vi "Acquire.vi"(8 "error in (no error)":errorcluster, 9 "Data Queue":refnum<queue>, 10 "Data Notifier":refnum<notifier>, 11 "Hardware Resources in":T1={"VISA resource name"="", "DAQ Type"=0, "Channel 1"={"Acquiring"=FALSE, "Enabled"=FALSE, "Terminal configuration"=32767, "Range"=0, "Coupling"=0}, "Channel 2"={"Acquiring"=FALSE, "Enabled"=FALSE, "Terminal configuration"=0, "Range"=0, "Coupling"=0}, "Timing"={"Sample Time [Time Units]"=0, "Actual Sample Time [s]"=0.0, "Samples per Iteration"=0, "Sample Clock Source"=0, "Time Units"=0, "t0"=timestamp(0 s since 1904-01-01), "Baud rate"=0}, "PS Parameters"={"PS handle"=0, "PS Max_adc"=32767, "PS Enabled Array"=[], "PS Device Info"={"Driver Version"="", "USB Version"="", "Hardware"="", "Variant"="", "Batch and Serial"="", "Cal Date"="", "Kernel Version"="", "Digital HW Version"="", "Analogue HW Version"="", "Firmware 1"="", "Firmware 2"="", "MSO"=FALSE, "Number of Channels"=0}, "Channel 1 Buffer"=refnum, "Channel 2 Buffer"=refnum, "Resolution"=0, "USB Power"=FALSE}, "Trigger"={"Direction"=0, "Threshold [V]"=0.0, "Enabled"=FALSE, "Trigger Source"=0}, "Keithley Parameters"={"Previous End / Current Start"=0, "Quantity"=0}} {"Keithley Parameters"."Quantity" items=["Current", "Voltage"]; "Trigger"."Trigger Source" items=["Channel 1"=0, "Channel 2"=1, "Ext."=4]; "Trigger"."Direction" items=["Falling", "Rising"]; "PS Parameters"."Resolution" items=["8", "12", "14", "15", "16"]; "Timing"."Time Units" items=["Seconds"]; "Timing"."Sample Clock Source" items=["Internal", "External"]; "Channel 2"."Coupling" items=["AC", "DC"]; "Channel 2"."Range" items=["0.01", "0.02", "0.05", "0.1", "0.2", "0.5", "1", "2", "5", "10", "20", "50", "100", "1000"]; "Channel 2"."Terminal configuration" items=["Referenced Single Ended", "Differential"]; "Channel 1"."Coupling" items=["AC", "DC"]; "Channel 1"."Range" items=["0.01", "0.02", "0.05", "0.1", "0.2", "0.5", "1", "2", "5", "10", "20", "50", "100", "1000"]; "Channel 1"."Terminal configuration" items=["Referenced Single Ended", "Differential"]; "DAQ Type" items=["Simulated", "Tektronics DPO2k/3k/4k", "PicoScope 2000a Series", "Keithley DMM7510", "PicoScope 5000a Series", "Arduino"]}) -> (0 "error out":errorcluster, 3 "Hardware Resources out":T1={"VISA resource name"="", "DAQ Type"=0, "Channel 1"={"Acquiring"=FALSE, "Enabled"=FALSE, "Terminal configuration"=32767, "Range"=0, "Coupling"=0}, "Channel 2"={"Acquiring"=FALSE, "Enabled"=FALSE, "Terminal configuration"=0, "Range"=0, "Coupling"=0}, "Timing"={"Sample Time [Time Units]"=0, "Actual Sample Time [s]"=0.0, "Samples per Iteration"=0, "Sample Clock Source"=0, "Time Units"=0, "t0"=timestamp(0 s since 1904-01-01), "Baud rate"=0}, "PS Parameters"={"PS handle"=0, "PS Max_adc"=32767, "PS Enabled Array"=[], "PS Device Info"={"Driver Version"="", "USB Version"="", "Hardware"="", "Variant"="", "Batch and Serial"="", "Cal Date"="", "Kernel Version"="", "Digital HW Version"="", "Analogue HW Version"="", "Firmware 1"="", "Firmware 2"="", "MSO"=FALSE, "Number of Channels"=0}, "Channel 1 Buffer"=refnum, "Channel 2 Buffer"=refnum, "Resolution"=0, "USB Power"=FALSE}, "Trigger"={"Direction"=0, "Threshold [V]"=0.0, "Enabled"=FALSE, "Trigger Source"=0}, "Keithley Parameters"={"Previous End / Current Start"=0, "Quantity"=0}} {"Keithley Parameters"."Quantity" items=["Current", "Voltage"]; "Trigger"."Trigger Source" items=["Channel 1"=0, "Channel 2"=1, "Ext."=4]; "Trigger"."Direction" items=["Falling", "Rising"]; "PS Parameters"."Resolution" items=["8", "12", "14", "15", "16"]; "Timing"."Time Units" items=["Seconds"]; "Timing"."Sample Clock Source" items=["Internal", "External"]; "Channel 2"."Coupling" items=["AC", "DC"]; "Channel 2"."Range" items=["0.01", "0.02", "0.05", "0.1", "0.2", "0.5", "1", "2", "5", "10", "20", "50", "100", "1000"]; "Channel 2"."Terminal configuration" items=["Referenced Single Ended", "Differential"]; "Channel 1"."Coupling" items=["AC", "DC"]; "Channel 1"."Range" items=["0.01", "0.02", "0.05", "0.1", "0.2", "0.5", "1", "2", "5", "10", "20", "50", "100", "1000"]; "Channel 1"."Terminal configuration" items=["Referenced Single Ended", "Differential"]; "DAQ Type" items=["Simulated", "Tektronics DPO2k/3k/4k", "PicoScope 2000a Series", "Keithley DMM7510", "PicoScope 5000a Series", "Arduino"]})   [LabVIEW 2017, in "Acquisition.lvlib"]
doc: "Perform the acquisition. Replace the contents of this diagram with calls to acquisition hardware."
uses:
  Acquisition.lvlib
  Hardware Configuration.ctl
  Signal Type.ctl
  Settings/Terminal Configuration.ctl
  Settings/Range.ctl
  Settings/Coupling.ctl
  Settings/Sampling Clock Source.ctl
  Settings/Time Units.ctl
  Settings/Resolution.ctl
  Settings/Trigger Direction.ctl
  Settings/Trigger Source.ctl
  Settings/Quantity.ctl
  support/Active channels.vi
  Settings/Settings.lvlib
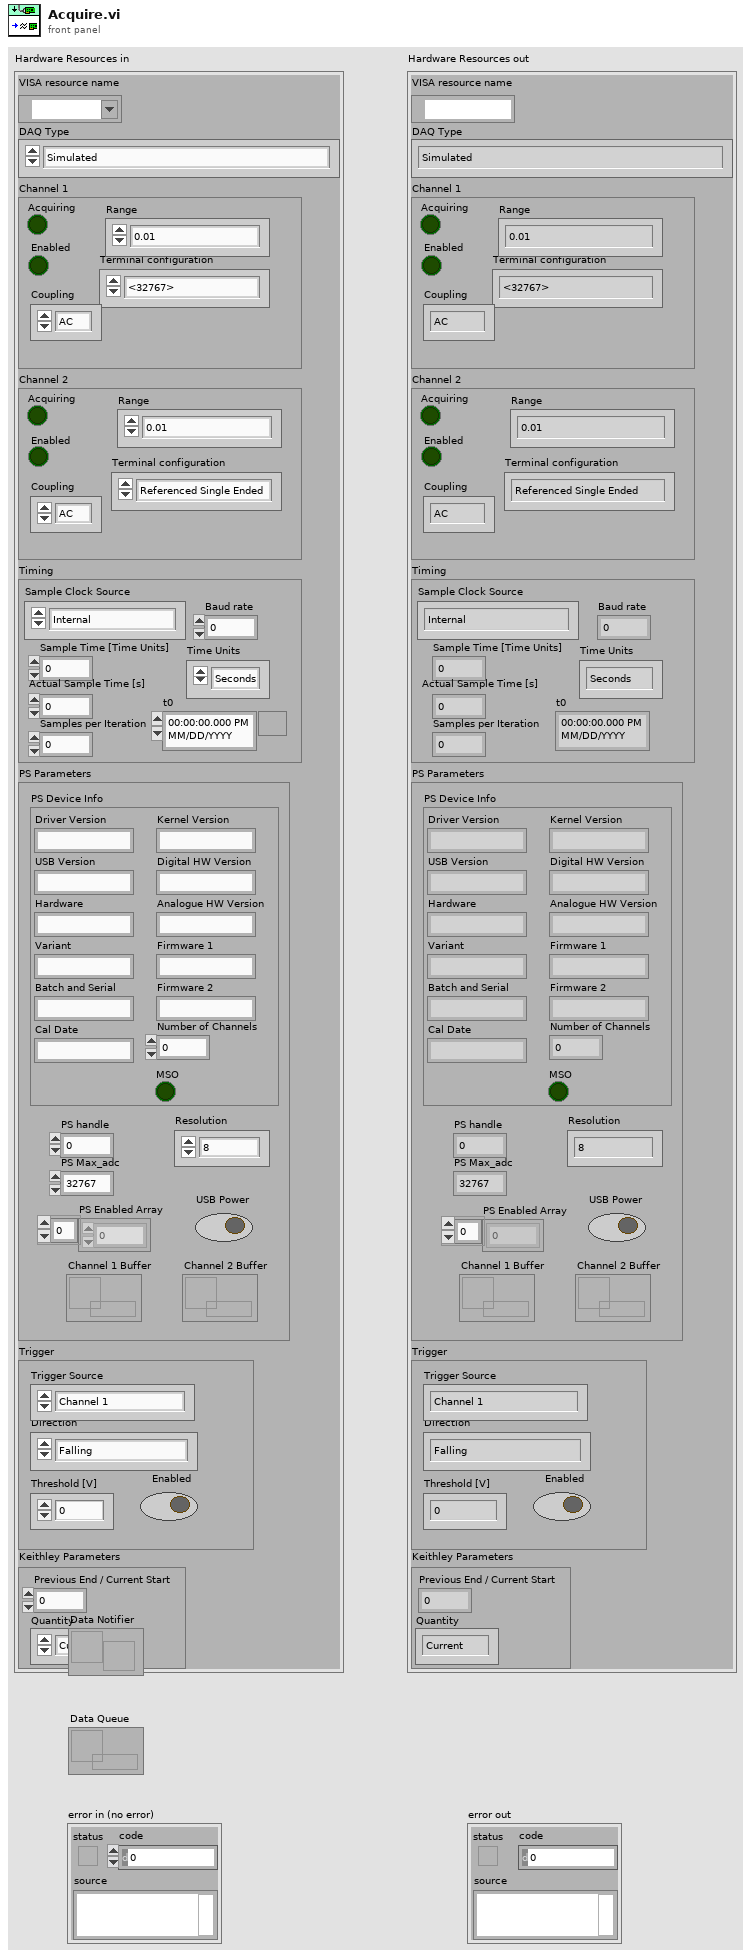
[diagram p1: front panel]
types:
  T1 = typedef "Acquisition.lvlib/Hardware Configuration.ctl" = cluster{"VISA resource name":refnum<visa-resource-name>, "DAQ Type":T2, "Channel 1":cluster{"Acquiring":bool, "Enabled":bool, "Terminal configuration":T3, "Range":T4, "Coupling":T5}, "Channel 2":cluster{"Acquiring":bool, "Enabled":bool, "Terminal configuration":T3, "Range":T4, "Coupling":T5}, "Timing":cluster{"Sample Time [Time Units]":u32, "Actual Sample Time [s]":dbl, "Samples per Iteration":u32, "Sample Clock Source":T6, "Time Units":T7, "t0":timestamp, "Baud rate":u32}, "PS Parameters":cluster{"PS handle":i16, "PS Max_adc":i16, "PS Enabled Array":i16[], "PS Device Info":cluster{"Driver Version":string, "USB Version":string, "Hardware":string, "Variant":string, "Batch and Serial":string, "Cal Date":string, "Kernel Version":string, "Digital HW Version":string, "Analogue HW Version":string, "Firmware 1":string, "Firmware 2":string, "MSO":bool, "Number of Channels":i16}, "Channel 1 Buffer":refnum<data-value>, "Channel 2 Buffer":refnum<data-value>, "Resolution":T8, "USB Power":bool}, "Trigger":cluster{"Direction":T9, "Threshold [V]":dbl, "Enabled":bool, "Trigger Source":T10}, "Keithley Parameters":cluster{"Previous End / Current Start":i32, "Quantity":T11}}
  T2 = typedef "Acquisition.lvlib/Signal Type.ctl" = u16
  T3 = typedef "Settings.lvlib/Terminal Configuration.ctl" = u16
  T4 = typedef "Settings.lvlib/Range.ctl" = u16
  T5 = typedef "Settings.lvlib/Coupling.ctl" = i16
  T6 = typedef "Settings.lvlib/Sampling Clock Source.ctl" = u16
  T7 = typedef "Settings.lvlib/Time Units.ctl" = u32
  T8 = typedef "Settings.lvlib/Resolution.ctl" = i32
  T9 = typedef "Settings.lvlib/Trigger Direction.ctl" = u16
  T10 = typedef "Settings.lvlib/Trigger Source.ctl" = u16
  T11 = typedef "Settings.lvlib/Quantity.ctl" = u16
  T12 = cluster{"PS handle":i16, "PS Max_adc":i16, "PS Enabled Array":i16[], "PS Device Info":cluster{"Driver Version":string, "USB Version":string, "Hardware":string, "Variant":string, "Batch and Serial":string, "Cal Date":string, "Kernel Version":string, "Digital HW Version":string, "Analogue HW Version":string, "Firmware 1":string, "Firmware 2":string, "MSO":bool, "Number of Channels":i16}, "Channel 1 Buffer":refnum<data-value>, "Channel 2 Buffer":refnum<data-value>, "Resolution":T8, "USB Power":bool}
  T13 = cluster{"Previous End / Current Start":i32, "Quantity":T11}
  T14 = cluster{"Acquiring":bool, "Enabled":bool, "Terminal configuration":T3, "Range":T4, "Coupling":T5}
  T15 = cluster{"Sample Time [Time Units]":u32, "Actual Sample Time [s]":dbl, "Samples per Iteration":u32, "Sample Clock Source":T6, "Time Units":T7, "t0":timestamp, "Baud rate":u32}
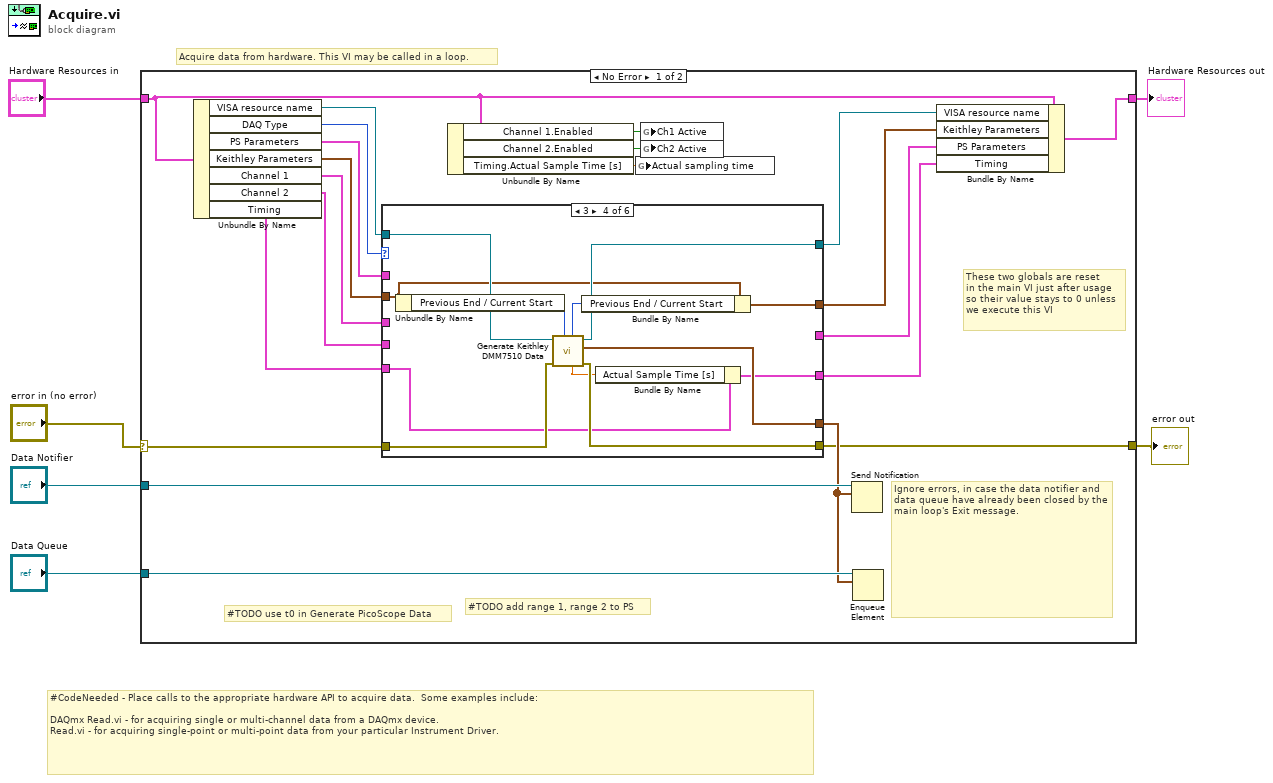
[diagram p0: block diagram]
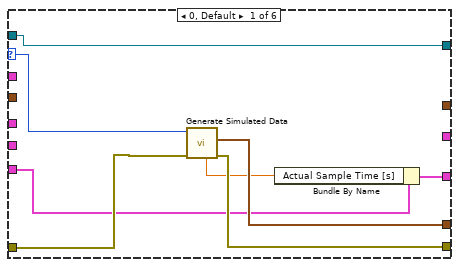
[diagram p2: hidden frame]
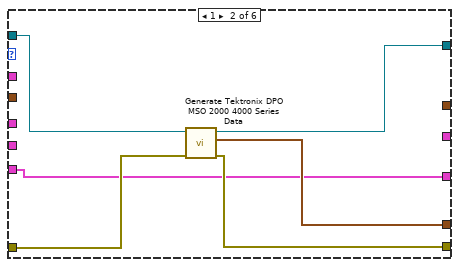
[diagram p3: hidden frame]
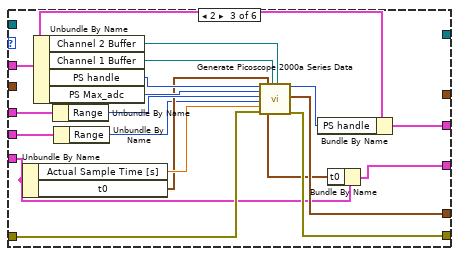
[diagram p4: hidden frame]
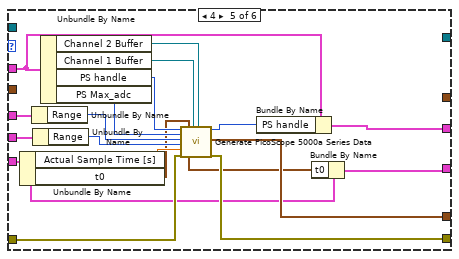
[diagram p5: hidden frame]
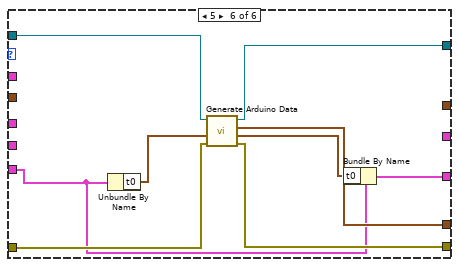
[diagram p6: hidden frame]
diagram:
  # "Acquire data from hardware. This VI may be called in a loop."
  # "#CodeNeeded - Place calls to the appropriate hardware API to acquire data.  Some examples include:\n\nDAQmx Read.vi - for acquiring single or multi-channel data from a DAQmx device.\nRead.vi - for acquiring single-point or multi-point data from your particular Instrument Driver."
  n1 = case shown="No Error" "error in (no error)" {
    selector: "error in (no error)" -> [w26 w101]
    tunnel: [w22 w101] -> w5
    tunnel: "Hardware Resources in" -> [w10 w102]
    tunnel: [w27 w102] -> w3
    tunnel: "Data Notifier" -> [w25 _]
    tunnel: "Data Queue" -> [w24 _]
    frame No Error {
      # "#TODO add range 1, range 2 to PS"
      # "These two globals are reset\nin the main VI just after usage\nso their value stays to 0 unless\nwe execute this VI"
      # "#TODO use t0 in Generate PicoScope Data"
      # "Ignore errors, in case the data notifier and data queue have already been closed by the main loop's Exit message."
      n2 = Unbundle By Name(w10) -> ("VISA resource name"=w20:refnum<visa-resource-name>, "DAQ Type"=w21:T2, "PS Parameters"=w15:T12, "Keithley Parameters"=w18:T13, "Channel 1"=w14:T14, "Channel 2"=w13:T14, "Timing"=w12:T15)
      n3 = case shown="3" w21 {
        selector: w21 -> [w31 _ _ _ _ _]
        tunnel: w26 -> [w34 w41 w59 w71 w91 w99]
        tunnel: [w32 w38 w55 w68 w89 w97] -> w23
        tunnel: [w33 w40 w58 w69 w90 w98] -> w22
        tunnel: w20 -> [w35 w39 _ w72 _ w100]
        tunnel: [w35 w37 _ w70 _ w96] -> w19
        tunnel: w18 -> [_ _ _ w66 _ _]
        tunnel: w15 -> [_ _ w57 _ w87 _]
        tunnel: w12 -> [w30 w36 w45 w63 w76 w93]
        tunnel: [_ _ w60 _ w85 _] -> w17
        tunnel: [_ _ _ w64 _ _] -> w16
        tunnel: w14 -> [_ _ w50 _ w80 _]
        tunnel: w13 -> [_ _ w49 _ w78 _]
        tunnel: [w29 w36 w43 w61 w75 w92] -> w11
        frame 0, Default {
          n4 = call "Generate Simulated Data.vi"("error in (no error)"=w34, "Signal Type"=w31) -> ("error out"=w33:errorcluster, "Graph Data"=w32:waveform(dbl)[], "Sampling time"=w28:dbl)  [unwired: 7 in]
          n5 = Bundle By Name(cluster=w30, "Actual Sample Time [s]"=w28) -> (w29:T15)
        }
        frame 1 {
          n6 = call "Generate Tektronix DPO MSO 2000 4000 Series Data.vi"("error in (no error)"=w41, "VISA resource name"=w39) -> ("error out"=w40:errorcluster, "Graph Data"=w38:waveform(dbl)[], "VISA resource name 2"=w37:refnum<visa-resource-name>)  [unwired: 7 in]
        }
        frame 2 {
          n7 = Unbundle By Name(w45) -> ("Actual Sample Time [s]"=w47:dbl, "t0"=w46:timestamp)
          n8 = Unbundle By Name(w57) -> ("Channel 2 Buffer"=w54:refnum<data-value>, "Channel 1 Buffer"=w53:refnum<data-value>, "PS handle"=w52:i16, "PS Max_adc"=w51:i16)
          n9 = Unbundle By Name(w50) -> ("Range"=w48:T4)
          n10 = Unbundle By Name(w49) -> ("Range"=w42:T4)
          n11 = call "Generate Picoscope 2000a Series Data.vi"("handle in"=w52, "Max ADC"=w51, "Ch1 Range Index"=w48, "Ch2 Range Index"=w42, "Actual Sample Interval"=w47, "error in (no error)"=w59, "t0"=w46, "Channel 1 Buff In"=w53, "Channel 2 Buff In"=w54) -> ("next t0"=w44:timestamp, "handle out"=w56:i16, "Graph Data"=w55:waveform(dbl)[], "error out"=w58:errorcluster)  [unwired: 5 in, 2 out]
          n12 = Bundle By Name(cluster=w57, "PS handle"=w56) -> (w60:T12)
          n13 = Bundle By Name(cluster=w45, "t0"=w44) -> (w43:T15)
        }
        frame 3 {
          n14 = Unbundle By Name(w66) -> ("Previous End / Current Start"=w67:i32)
          n15 = call "Generate Keithley DMM7510 Data.vi"("Previous End"=w67, "error in (no error)"=w71, "VISA resource name in"=w72) -> ("error out"=w69:errorcluster, "Graph Data"=w68:waveform(dbl)[], "VISA resource name out"=w70:refnum<visa-resource-name>, "Actual sampling time (mean)"=w62:dbl, "Current End"=w65:i32)  [unwired: 4 in]
          n16 = Bundle By Name(cluster=w66, "Previous End / Current Start"=w65) -> (w64:T13)
          n17 = Bundle By Name(cluster=w63, "Actual Sample Time [s]"=w62) -> (w61:T15)
        }
        frame 4 {
          n18 = Unbundle By Name(w76) -> ("Actual Sample Time [s]"=w88:dbl, "t0"=w74:timestamp)
          n19 = Unbundle By Name(w80) -> ("Range"=w79:T4)
          n20 = Unbundle By Name(w78) -> ("Range"=w77:T4)
          n21 = Unbundle By Name(w87) -> ("Channel 2 Buffer"=w83:refnum<data-value>, "Channel 1 Buffer"=w84:refnum<data-value>, "PS handle"=w82:i16, "PS Max_adc"=w81:i16)
          n22 = call "Generate PicoScope 5000a Series Data.vi"("handle in"=w82, "Max ADC"=w81, "Ch1 Range Index"=w79, "Ch2 Range Index"=w77, "Actual Sample Interval"=w88, "error in (no error)"=w91, "t0"=w74, "Channel 1 Buff In"=w84, "Channel 2 Buff In"=w83) -> ("next t0"=w73:timestamp, "handle out"=w86:i16, "Graph Data"=w89:waveform(dbl)[], "error out"=w90:errorcluster)  [unwired: 5 in, 2 out]
          n23 = Bundle By Name(cluster=w87, "PS handle"=w86) -> (w85:T12)
          n24 = Bundle By Name(cluster=w76, "t0"=w73) -> (w75:T15)
        }
        frame 5 {
          n25 = Unbundle By Name(w93) -> ("t0"=w95:timestamp)
          n26 = call "Generate Arduino Data.vi"("error in (no error)"=w99, "t0"=w95, "VISA resource name in"=w100) -> ("error out"=w98:errorcluster, "next t0"=w94:timestamp, "Graph Data"=w97:waveform(dbl)[], "VISA resource name out"=w96:refnum<visa-resource-name>)  [unwired: 5 in]
          n27 = Bundle By Name(cluster=w93, "t0"=w94) -> (w92:T15)
        }
      }
      n28 = Unbundle By Name(w10) -> ("Channel 1.Enabled"=w9:bool, "Channel 2.Enabled"=w7:bool, "Timing.Actual Sample Time [s]"=w8:dbl)
      n29 = global write "Active channels.vi" "Actual sampling time"(w8) -> ()
      n30 = global write "Active channels.vi" "Ch1 Active"(w9) -> ()
      n31 = global write "Active channels.vi" "Ch2 Active"(w7) -> ()
      n32 = Send Notification(notification=w23, notifier=w25) -> ()  [unwired: 1 in, 2 out]
      n33 = Enqueue Element(queue=w24, element=w23) -> ()  [unwired: 2 in, 3 out]
      n34 = Bundle By Name(cluster=w10, "VISA resource name"=w19, "Keithley Parameters"=w16, "PS Parameters"=w17, "Timing"=w11) -> (w27:T1)
    }
    frame Error {
    }
  }
  "Hardware Resources out" <- w3
  "error out" <- w5
